vi "MandM.vi"(0 "ROI Descriptor (Color Location 1)":T1={"Global Rectangle"=[388, 602, 2797, 2374], "Contours"=[{"ID"=enum."External", "Type"=12, "Coordinates"=[388, 602, 2797, 2374, 0]}]} {"Contours"."Type" items=["No Selection", "Point", "Line", "Rectangle", "Oval", "Polygon", "Freehand Region", "Annulus", "Unused2", "Unused3", "Broken Line", "Freehand Line", "Rotated Rectangle"]}, 1 "Number of Matches Requested (Color Location 1)":i32=11, 2 "Minimum Match Score (Color Location 1)":sgl=800.0, 7 "error in":errorcluster) -> (20 "Matches (Color Location 1)":T3(array[cluster]) {"Bounding Box"."y" format="%.2f"; "Bounding Box"."x" format="%.2f"; "Position"."y" format="%.2f"; "Position"."x" format="%.2f"; "Score" format="%.2f"; "Scale" format="%.2f"; "Angle" format="%.2f"}, 21 "Number of Matches (Color Location 1)":i32, 27 "error out":errorcluster)   [LabVIEW 2015]
uses:
  <vilib>/vision/NI_Vision_Development_Module.lvlib
panel:
  out "Image Out":T2(plugin-control)
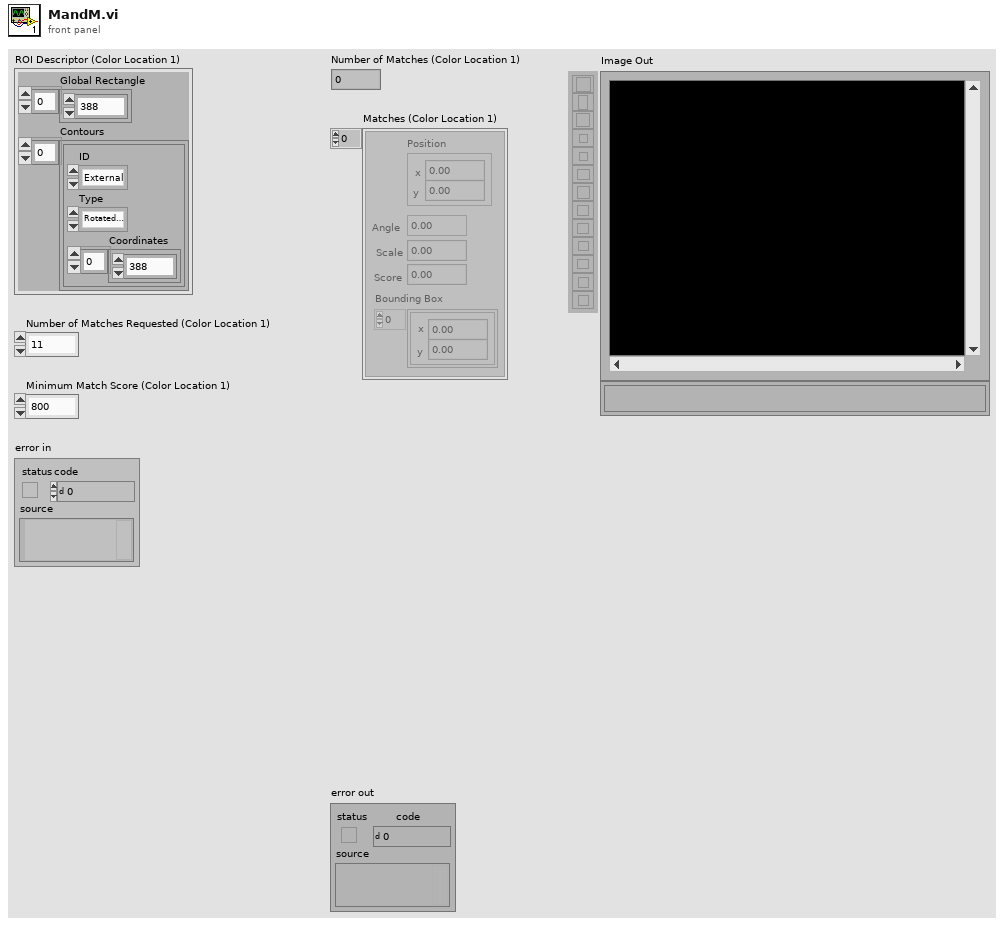
[diagram p1: front panel]
types:
  T1 = cluster{"Global Rectangle":i32[], "Contours":cluster{"ID":enum32{"External", "Internal"}, "Type":u32, "Coordinates":i32[]}[]}
  T2 = typedef "IMAQ Image.ctl" = refnum<image>
  T3 = cluster{"Position":cluster{"x":sgl, "y":sgl}, "Angle":sgl, "Scale":sgl, "Score":sgl, "Bounding Box":cluster{"x":sgl, "y":sgl}[]}[]
  T4 = typedef "Image Type" = u32
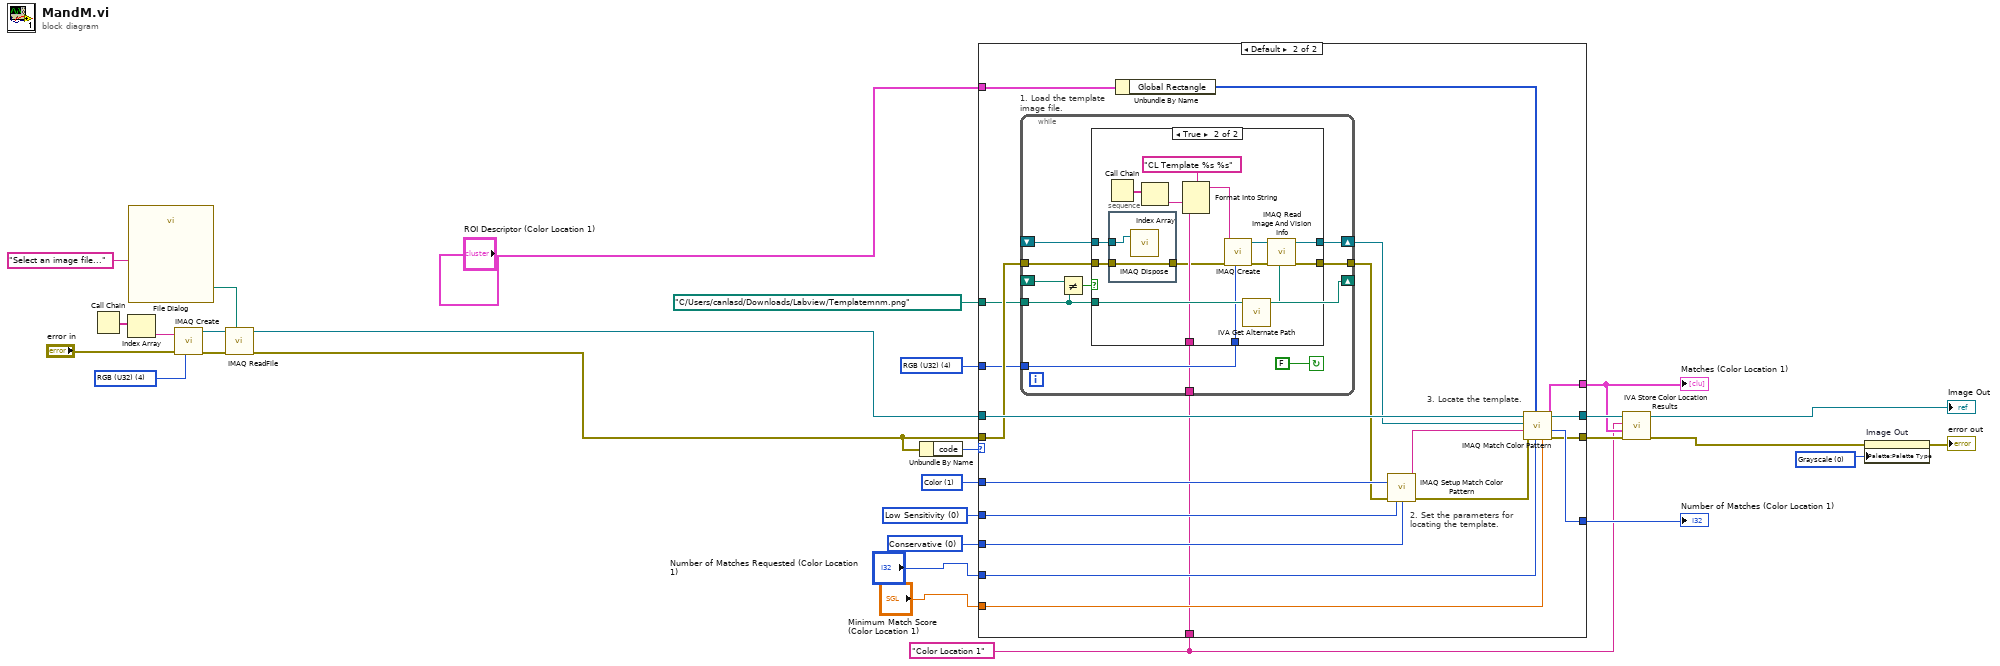
[diagram p0: block diagram]
diagram:
  w1 = u32 0 items=["Grayscale", "Binary", "Gradient", "Rainbow", "Temperature", "User Defined", "Binary 16 Bit", "Gradient 16 Bit", "Rainbow 16 Bit", "Temperature 16 Bit", "User Defined 16 Bit"] ("Palette Type")
  w4 = "Color Location 1" ("Step Name")
  w12 = T4 4 items=["Grayscale (U8)", "Grayscale (I16)", "Grayscale (SGL)", "Complex (CSG)", "RGB (U32)", "HSL (U32)", "RGB (U64)"] ("Image Type")
  w14 = u32 0 items=["Conservative", "Balance", "Aggressive", "Very Aggressive"] ("Search Strategy")
  w15 = u32 0 items=["Low Sensitivity", "Medium Sensitivity", "High Sensitivity"] ("Color Sensitivity")
  w16 = u32 1 items=["Color and Shape", "Color", "Shape"] ("Match Feature Mode")
  w20 = T4 4 items=["Grayscale (U8)", "Grayscale (I16)", "Grayscale (SGL)", "Complex (CSG)", "RGB (U32)", "HSL (U32)", "RGB (U64)", "Grayscale (U16)"] ("Image Type")
  n1 = Call Chain() -> (call chain=w24:string[])
  n2 = Index Array(array=w24) -> (element=w23:string)  [unwired: 1 in]
  n3 = call "File Dialog"("prompt"="Select an image file...") -> ("selected path"=w21:path)  [unwired: 6 in, 8 out]
  n4 = call "IMAQ Create"("Image Name"=w23, "Image Type"=w20, "error in (no error)"="error in") -> ("New Image"=w27:T2, "error out"=w26:errorcluster)  [unwired: 1 in, 1 out]
  n5 = call "IMAQ ReadFile"("File Path"=w21, "error in (no error)"=w26, "Image"=w27) -> ("error out"=w28:errorcluster, "Image Out"=w10:T2)  [unwired: 2 in, 5 out]
  n6 = Unbundle By Name(w28) -> ("code"=w9:i32)
  n7 = case shown="Default" w9 {
    tunnel: "Minimum Match Score (Color Location 1)" -> [_ w48]
    tunnel: "Number of Matches Requested (Color Location 1)" -> [_ w47]
    tunnel: [_ w46] -> w17
    tunnel: w16 -> [_ w45]
    tunnel: w15 -> [_ w44]
    tunnel: w14 -> [_ w43]
    tunnel: path "C:/Users/canlasd/Downloads/Labview/Templatemnm.png" ("File Path") -> [_ w35]
    tunnel: w12 -> [_ w34]
    tunnel: w28 -> [_ w36]
    tunnel: "ROI Descriptor (Color Location 1)" -> [_ w40]
    tunnel: [_ w38] -> w5
    tunnel: w10 -> [w29 w37]
    tunnel: [w29 w37] -> w6
    tunnel: [_ w31] -> w7
    tunnel: w4 -> [_ w30]
    frame -1074396199, -1074396198 {
      # "Discard Coordinate System Error"
    }
    frame Default {
      # "3. Locate the template."
      # "2. Set the parameters for\nlocating the template."
      n8 = while "1. Load the template image file." {
        shift-right: [w58] -> w33
        shift-left: _ -> [w57]
        tunnel: [w55] -> w32
        tunnel: w36 -> [w54]
        tunnel: w35 -> [w49]
        tunnel: w34 -> [w53]
        tunnel: w30 -> [w52]
        shift-right: [w49] -> _
        shift-left: _ -> [w51]
        stop <- FALSE continue-if-true
        n9 = Not Equal?(x=w51, y=w49) -> (x != y?=w50:bool)
        n10 = case shown="True" w50 {
          tunnel: [w60 w73] -> w58
          tunnel: w57 -> [w60 w65]
          tunnel: [w59 w70] -> w55
          tunnel: w54 -> [w59 w64]
          tunnel: w53 -> [_ w69]
          tunnel: w52 -> [_ w66]
          tunnel: w49 -> [_ w62]
          frame False {
          }
          frame True {
            n11 = Call Chain() -> (call chain=w68:string[])
            n12 = stacked-sequence {
              tunnel: w65 -> [w77]
              tunnel: w64 -> [w76]
              tunnel: [w76] -> w63
              frame #0 {
                n13 = call "IMAQ Dispose"("Image"=w77) -> ()  [unwired: 2 in, 4 out]
              }
            }
            n14 = Index Array(array=w68) -> (element=w67:string)  [unwired: 1 in]
            n15 = Format Into String(format string="CL Template %s %s" ("Image Name"), w67, w66) -> (resulting string=w75:string)  [unwired: 2 in, 1 out]
            n16 = call "IMAQ Create"("Image Name"=w75, "Image Type"=w69, "error in (no error)"=w63) -> ("New Image"=w72:T2, "error out"=w71:errorcluster)  [unwired: 1 in, 1 out]
            n17 = call <vilib>:"IVA Get Alternate Path.vi"("Path In"=w62) -> ("Path Out"=w61:path)  [unwired: 10 out]
            n18 = call "IMAQ Read Image And Vision Info"("File Path"=w61, "error in (no error)"=w71, "Image"=w72) -> ("error out"=w70:errorcluster, "Image Out"=w73:T2)  [unwired: 1 in, 6 out]
          }
        }
      }
      n19 = Unbundle By Name(w40) -> ("Global Rectangle"=w39:i32[])
      n20 = call "IMAQ Setup Match Color Pattern"("Match Feature Mode"=w45, "error in (no error)"=w32, "Color Sensitivity"=w44, "Search Strategy"=w43) -> ("Match Color Pattern Setup Data"=w42:string, "error out"=w41:errorcluster)  [unwired: 5 in, 5 out]
      n21 = call "IMAQ Match Color Pattern"("Minimum Match Score"=w48, "Number of Matches Requested"=w47, "Optional Rectangle"=w39, "error in (no error)"=w41, "Match Color Pattern Setup Data"=w42, "Template Image"=w33, "Image"=w37) -> ("error out"=w31:errorcluster, "Number of Matches"=w46:i32, "Matches"=w38:T3)  [unwired: 2 out]
    }
  }
  "Number of Matches (Color Location 1)" <- w17
  "Matches (Color Location 1)" <- w5
  n22 = call <vilib>:"IVA Store Color Location Results.vi"("error in (no error)"=w7, "Matches"=w5, "Step Name"=w4, "Image in"=w6) -> ("error out"=w8:errorcluster, "Image dup"=→"Image Out":T2)  [unwired: 6 out]
  n23 = property on="Image Out" class="ImageControl"(error in=w8, "Palette:Palette Type"=w1) -> (error out=→"error out":errorcluster)  [unwired: 1 in, 1 out]
